vi "dfd_DFXP_DFXP to Extended (scaler).vi"(11 "Value in":T1 {"Low 64" format="%.0x"; "High 64" format="%.0x"}) -> (3 "Ext value":ext)   [LabVIEW 2017, in "NI_DigFilter_FXP.lvlib"]
uses:
  <vilib>/addons/Digital Filter Design/NI_DigFilter_FXP.lvlib
  <vilib>/addons/Digital Filter Design/_Objects.llb/dfd_DFXP Data Type 128bits (scaler).ctl
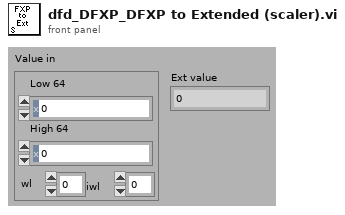
[diagram p1: front panel]
types:
  T1 = typedef "dfd_DFXP Data Type 128bits (scaler).ctl" = cluster{"Low 64":u64, "High 64":i64, "wl":i16, "iwl":i16}
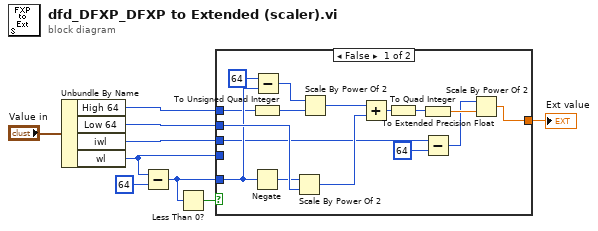
[diagram p0: block diagram]
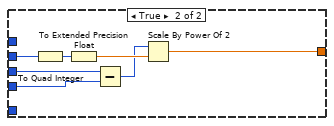
[diagram p2: hidden frame]
diagram:
  n1 = Unbundle By Name("Value in") -> ("High 64"=w2:i64, "Low 64"=w7:u64, "iwl"=w5:i16, "wl"=w6:i16)
  n2 = Subtract(x=w6, y=i16 64) -> (x-y=w3:i16)
  n3 = Less Than 0?(x=w3) -> (x < 0?=w4:bool)
  n4 = case shown="False" w4 {
    tunnel: w7 -> [w25 w31]
    tunnel: w6 -> [_ w29]
    tunnel: w5 -> [w15 w30]
    tunnel: [w13 w27] -> w1
    tunnel: w3 -> [w22 _]
    tunnel: w2 -> [w20 _]
    frame False {
      n5 = To Unsigned Quad Integer(1:w20) -> (0:w10:u64)
      n6 = Negate(x=w22) -> (-x=w24:i16)
      n7 = Subtract(x=i16 64 ("y"), y=w22) -> (x-y=w21:i16)
      n8 = Scale By Power Of 2(n=w24, x=w25) -> (x*2^n=w19:u64)
      n9 = Scale By Power Of 2(n=w21, x=w10) -> (x*2^n=w11:u64)
      n10 = Add(x=w11, y=w19) -> (x+y=w16:u64)
      n11 = To Quad Integer(1:w16) -> (0:w12:i64)
      n12 = To Extended Precision Float(1:w12) -> (0:w18:ext)
      n13 = Subtract(x=w15, y=i16 64) -> (x-y=w17:i16)
      n14 = Scale By Power Of 2(n=w17, x=w18) -> (x*2^n=w13:ext)
    }
    frame True {
      n15 = To Quad Integer(1:w31) -> (0:w26:i64)
      n16 = To Extended Precision Float(1:w26) -> (0:w32:ext)
      n17 = Subtract(x=w30, y=w29) -> (x-y=w28:i16)
      n18 = Scale By Power Of 2(n=w28, x=w32) -> (x*2^n=w27:ext)
    }
  }
  "Ext value" <- w1
